vi "LAC Cont Read (SubVI).vi"(7 "timeout(ms)":u32, 8 "error in":errorcluster, 11 "VISA name in":refnum<visa-resource-name>) -> (0 "error out":errorcluster, 1 "read buffer":string, 3 "VISA name out":refnum<visa-resource-name>)   [LabVIEW 8.6]
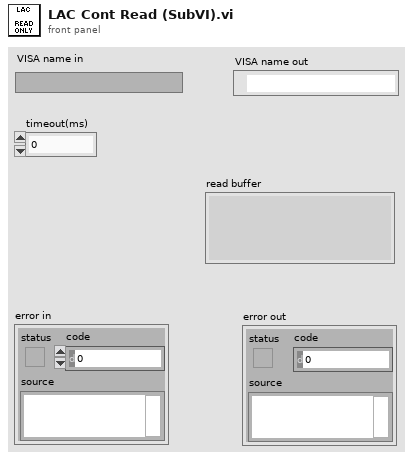
[diagram p1: front panel]
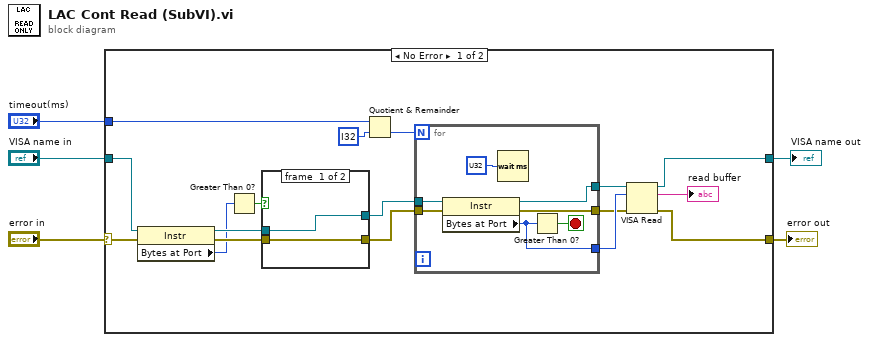
[diagram p0: block diagram]
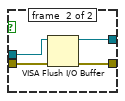
[diagram p2: hidden frame]
diagram:
  n1 = case shown="No Error" "error in" {
    selector: "error in" -> [w6 w37]
    tunnel: "VISA name in" -> [w7 w36]
    tunnel: [w18 w36] -> w4
    tunnel: [w16 w37] -> w3
    tunnel: "timeout(ms)" -> [w15 _]
    frame #0 {
      n2 = property class="Instr"(reference=w7, error in=w6) -> (reference out=w12:refnum<visa-resource-name>, error out=w13:errorcluster, "Bytes at Port"=w10:u32)
      n3 = Greater Than 0?(x=w10) -> (x > 0?=w11:bool)
      n4 = case shown="True" w11 {
        tunnel: w12 -> [w24 w26]
        tunnel: [w24 w25] -> w8
        tunnel: w13 -> [w23 w28]
        tunnel: [w23 w27] -> w9
        frame #0 {
        }
        frame #1 {
          n5 = VISA Flush I/O Buffer(VISA resource name=w26, error in (no error)=w28) -> (VISA resource name out=w25:refnum<visa-resource-name>, error out=w27:errorcluster)  [unwired: 1 in]
        }
      }
      n6 = Quotient & Remainder(x=w15, y=i32 ?) -> (floor(x/y)=w19:u32)  [unwired: 1 out]
      n7 = for {
        N: w19 -> [_]
        tunnel: w8 -> [w33]
        tunnel: [w31] -> w22
        tunnel: [w32] -> w21
        tunnel: w9 -> [w30]
        tunnel: [w29] -> w17
        stop <- w35 stop-if-true
        n8 = property class="Instr"(reference=w33, error in=w30) -> (reference out=w32:refnum<visa-resource-name>, error out=w29:errorcluster, "Bytes at Port"=w31:u32)
        n9 = Wait (ms)(milliseconds to wait=u32 ?) -> ()  [unwired: 1 out]
        n10 = Greater Than 0?(x=w31) -> (x > 0?=w35:bool)
      }
      n11 = VISA Read(VISA resource name=w21, byte count=w22, error in (no error)=w17) -> (VISA resource name out=w18:refnum<visa-resource-name>, read buffer=→"read buffer":string, error out=w16:errorcluster)  [unwired: 1 out]
    }
    frame #1 {
    }
  }
  "VISA name out" <- w4
  "error out" <- w3
